vi "Read Spectrum Notifier.vi"(8 "error in (no error)":errorcluster) -> (0 "error out":errorcluster, 2 "timed out?":bool, 3 "WaveForm Out":waveform(dbl))   [LabVIEW 2016]
doc: "Checks if there is data available in the spectrum data notifier."
uses:
  Application Control/Application Globals.vi
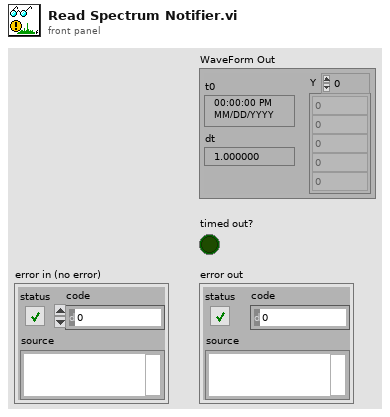
[diagram p1: front panel]
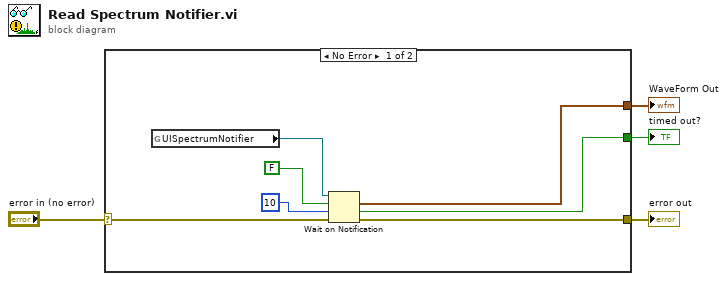
[diagram p0: block diagram]
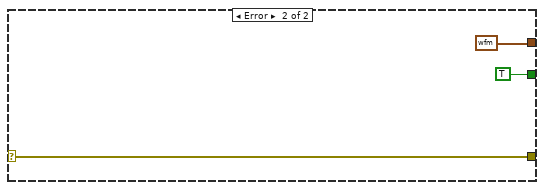
[diagram p2: hidden frame]
diagram:
  n1 = case shown="No Error" "error in (no error)" {
    selector: "error in (no error)" -> [w5 w14]
    tunnel: [w8 w14] -> w4
    tunnel: [w7 TRUE ("timed out?")] -> w3
    tunnel: [w6 waveform(dbl) {"t0"=timestamp(0 s since 1904-01-01), "dt"=1.0, "Y"=[]} ("data out")] -> w2
    frame No Error {
      n2 = global read "Application Globals.vi" "UISpectrumNotifier"() -> (w9:refnum<notifier>)
      n3 = Wait on Notification(notifier=w9, ignore previous (F)=FALSE, timeout in ms (-1)=10, error in (no error)=w5) -> (notification=w6:waveform(dbl), timed out?=w7:bool, error out=w8:errorcluster)  [unwired: 1 out]
    }
    frame Error {
    }
  }
  "error out" <- w4
  "timed out?" <- w3
  "WaveForm Out" <- w2
